vi "Teleop.vi"(10 "Match Info":T2={"Autonomous Elapsed Seconds"=0.0, "TeleOp Elapsed Seconds"=0.0, "Disabled Elapsed Seconds"=0.0, "Visited Autonomous"=FALSE, "Visited TeleOp"=FALSE, "Visited Disabled"=FALSE, "Autonomous Settings"={"Autonomous Style"=enum."Independent", "VI Refnum"=refnum}}, 11 "Call Context":T3) -> ()   [LabVIEW 2016]
doc: "This VI is called for each TeleOp packet received from the DS where the robot is not disabled. It is often used to read from the joysticks and update I/O or to update setpoints for timed control loops. It should complete and return within 20 milliseconds or it may miss DS packets."
uses:
  <vilib>/Rock Robotics/WPI/DriverStation/WPI_DriverStationDerivedRobotMode.ctl
  <vilib>/Rock Robotics/WPI/DriverStation/WPI_DriverStationMatch Info.ctl
  <vilib>/Rock Robotics/WPI/ThirdParty/CanMotor/TalonSRX/WPI_CANTalonSRX_BrakeOverride.ctl
  <vilib>/Rock Robotics/WPI/Utilities/WPI_GetSetVariantRefNum.vi
  <vilib>/Rock Robotics/Network Tables/NT Write Boolean Array.vi
  <vilib>/Rock Robotics/Network Tables/NT Write Numeric Array.vi
  <vilib>/Rock Robotics/Network Tables/NT Read Boolean.vi
  <vilib>/Rock Robotics/Network Tables/NT Read Number.vi
panel:
  in  "Output":dbl=0.5 format="%#_13g"
  in  "Reverse Soft Limit 2":dbl
  in  "Forward Soft Limit  2":dbl
  in  "Voltage Ramp Rate":dbl
  in  "Brake / Coast Mode":T1
  out "Brake Enabled":bool
  out "Reverse Soft Limit":bool
  out "Forward Soft Limit":bool
  out "Encoder V":dbl
  out "Battery Voltage":dbl
  out "Current":dbl
  out "Applied Throttle":dbl
  out "Sample Slider 0":dbl(slide) scale=0.0..5.0
  out "Sample Boolean 1":bool
  out "Sample Boolean 0":bool
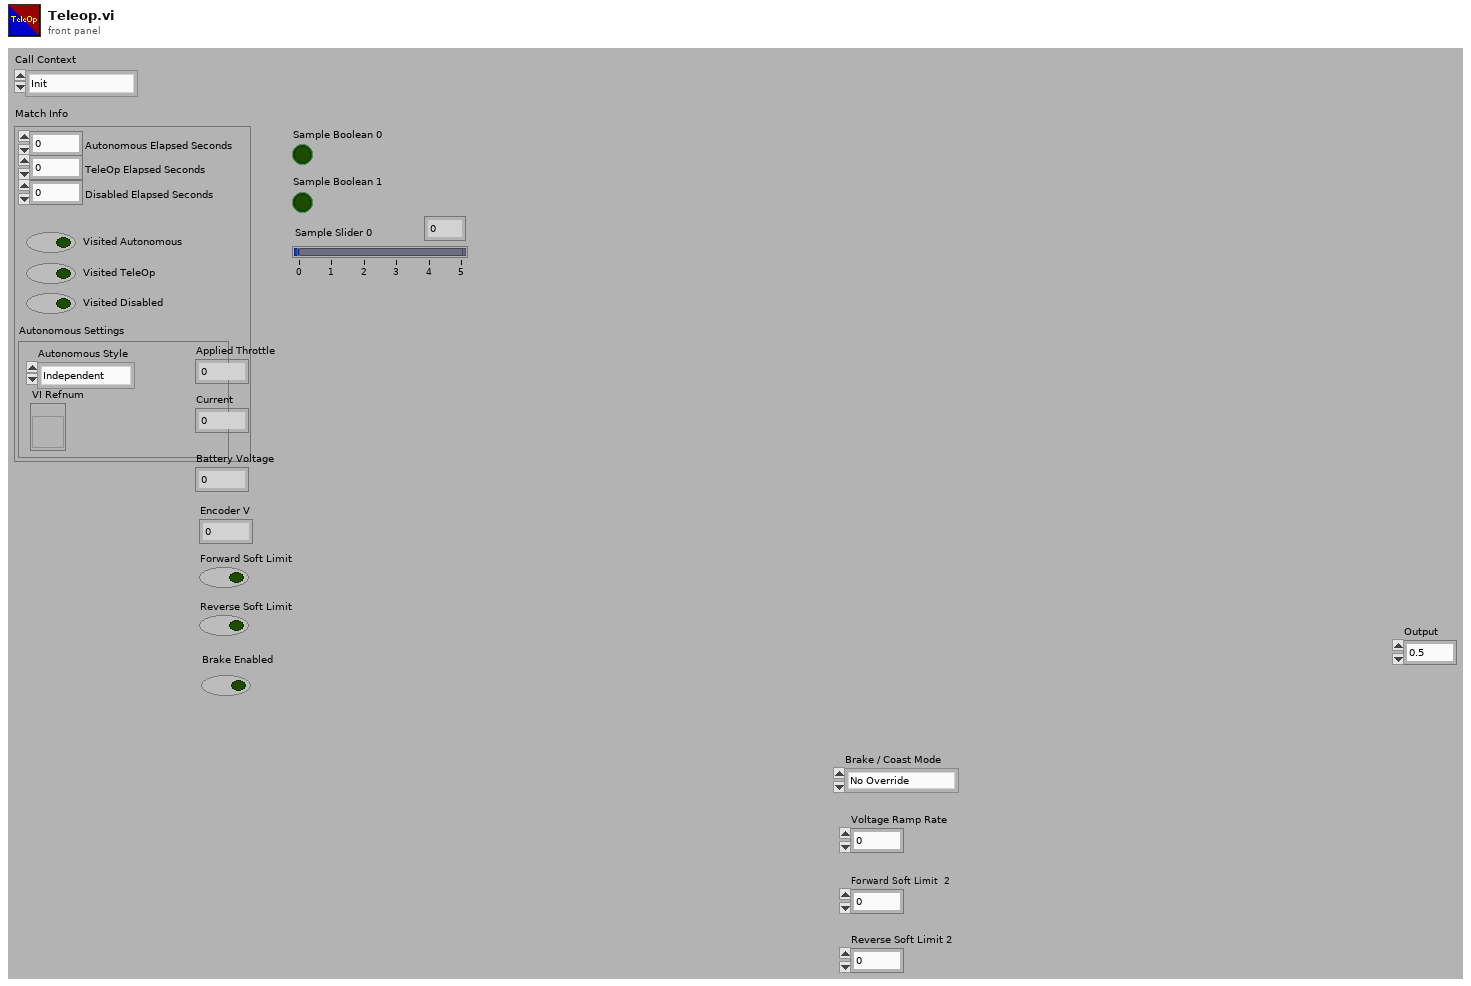
[diagram p1: front panel]
types:
  T1 = typedef "WPI_CANTalonSRX_BrakeOverride.ctl" = enum8{"No Override", "Override to Coast", "Override to Brake"}
  T2 = typedef "WPI_DriverStationMatch Info.ctl" = cluster{"Autonomous Elapsed Seconds":dbl, "TeleOp Elapsed Seconds":dbl, "Disabled Elapsed Seconds":dbl, "Visited Autonomous":bool, "Visited TeleOp":bool, "Visited Disabled":bool, "Autonomous Settings":cluster{"Autonomous Style":enum16{"Iterative", "Independent"}, "VI Refnum":refnum<vi>}}
  T3 = typedef "WPI_DriverStationDerivedRobotMode.ctl" = enum16{"Init", "Execute", "Stop"}
  T4 = typedef "WPI_RobotDriveDevRef.ctl" = cluster{"DevStatus":errorcluster, "Motors[]":T5[], "Square Inputs":bool, "Max Output":dbl}
  T5 = typedef "WPI_MotorControlDeviceRef.ctl" = cluster{"DeviceStatus":errorcluster, "Type":T6, "PWM":cluster{"PWM Channel":T7, "DeadBand":T8}, "CAN":cluster{"Device Number":u8, "SetOutput VI Ref":variant, "GetOutput VI Ref":variant, "Enable VI Ref":variant, "Disable VI Ref":variant, "Data":variant}, "Invert":bool}
  T6 = typedef "WPI_MotorControlType.ctl" = enum16{"PWM", "CAN"}
  T7 = typedef "FPGA_DIOPWMChannel.ctl" = enum8{"PWM 0", "PWM 1", "PWM 2", "PWM 3", "PWM 4", "PWM 5", "PWM 6", "PWM 7", "PWM 8", "PWM 9", "PWM MXP 0", "PWM MXP 1", "PWM MXP 2", "PWM MXP 3", "PWM MXP 4", "PWM MXP 5", "PWM MXP 6", "PWM MXP 7", "PWM MXP 8", "PWM MXP 9", "Invalid"}
  T8 = typedef "WPI_PWMDeadband.ctl" = cluster{"Name":string, "maxPositivePwm":i32, "minPositivePwm":i32, "centerPwm":i32, "maxNegativePwm":i32, "minNegativePwm":i32, "angularRange":u16}
  T9 = typedef "WPI_JoystickDevRef.ctl" = cluster{"Device":T10}
  T10 = typedef "WPI_JoystickDeviceEnum.ctl" = enum16{"USB 0", "USB 1", "USB 2", "USB 3", "USB 4", "USB 5"}
  T11 = typedef "WPI_CANTalonSRX_GlobalStatus.ctl" = cluster{"Applied Throttle":dbl, "Module Enabled":bool, "CAN Error":errorcluster, "Closed Loop Error":dbl, "Forward Limit Switch Closed":bool, "Reverse Limit Switch Closed":bool, "Sensor Position":dbl, "Sensor Velocity":dbl, "Current":dbl, "Sticky Fault - Over Temp":bool, "Sticky Fault - Under Voltage":bool, "Sticky Fault - Forward Limit":bool, "Sticky Fault - Reverse Limit":bool, "Sticky Fault - Forward Soft Limit":bool, "Sticky Fault - Reverse Soft Limit":bool, "Brake is Enabled":bool, "Encoder Position":dbl, "Encoder Velocity":dbl, "Encoder Index Count":dbl, "Encoder A Pin State":bool, "Encoder B Pin State":bool, "Encoder Index Pin State":bool, "Analog In":dbl, "Analog In Velocity":dbl, "Temperature (C)":dbl, "Battery Voltage":dbl, "Control 5 Is Supported":bool, "Current Profile Slot Select":dbl, "Pos Div 8":bool, "Vel Div 4":bool, "Pulse Width Position":i32, "Pulse Width Velocity":i32, "Pulse Width Rise To Rise (us)":i32, "Pulse Width Rise To Fall (us)":i32, "Mot Prof Active Is Under Run":bool, "Mot Prof Active Has Under Run":bool, "Mot Prof Active Is Last":bool, "Mot Prof Active Velocity Only":bool, "Mot Prof Active Is Valid":bool, "Mot Prof Buffer Is Full":bool, "Mot Prof Active Profile Slot Select":i32, "Mot Prof NextID":i32, "Mot Prof Count":i32, "Mot Prof Active Velocity":dbl, "Mot Prof Active Position":dbl, "Mot Prof Output Enable":i32}
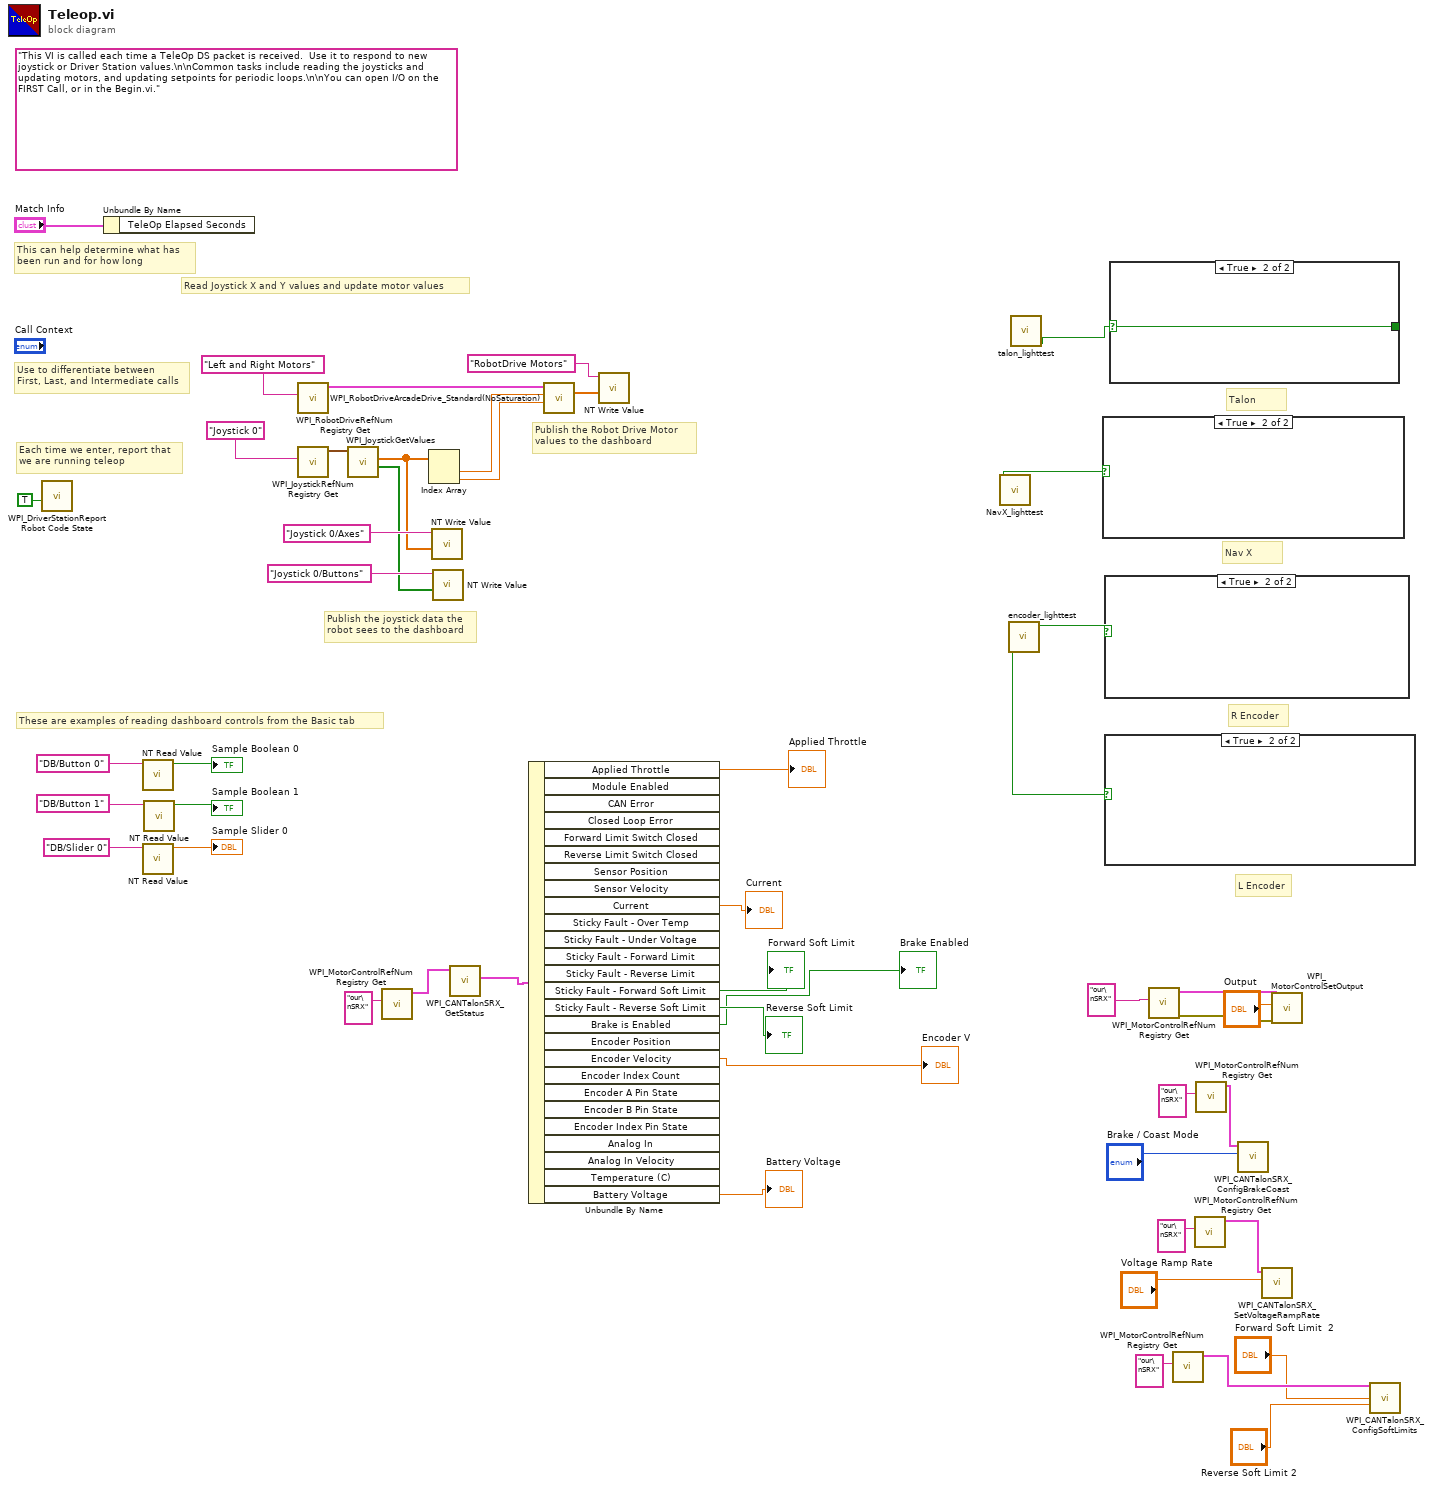
[diagram p0: block diagram]
diagram:
  (unwired) "This VI is called each time a TeleOp DS packet is received.  Use it to respond to new joystick or Driver Station values.\n\nCommon tasks include reading the joysticks and updating motors, and updating setpoints for periodic loops.\n\nYou can open I/O on the FIRST Call, or in the Begin.vi."
  # "Talon"
  # "Nav X"
  # "R Encoder"
  # "L Encoder"
  # "These are examples of reading dashboard controls from the Basic tab"
  # "Publish the Robot Drive Motor\nvalues to the dashboard"
  # "Publish the joystick data the\nrobot sees to the dashboard"
  # "Each time we enter, report that\nwe are running teleop"
  # "Use to differentiate between\nFirst, Last, and Intermediate calls"
  # "This can help determine what has\nbeen run and for how long"
  # "Read Joystick X and Y values and update motor values"
  n1 = call <vilib>:"WPI_DriverStationReport Robot Code State.vi"("TeleOp"=TRUE ("Autonomous")) -> ()  [unwired: 10 in, 1 out]
  n2 = Unbundle By Name("Match Info") -> ()  [unwired: 1 out]
  n3 = call-poly <vilib>:"NT Read Value.vi"("Name"="DB/Button 0" ("refnum name")) -> ("Boolean"=→"Sample Boolean 0":bool)  [unwired: 9 in, 1 out]
  n4 = call-poly <vilib>:"NT Read Value.vi"("Name"="DB/Slider 0" ("refnum name")) -> ("Numeric"=→"Sample Slider 0":dbl)  [unwired: 9 in, 1 out]
  n5 = call-poly <vilib>:"NT Read Value.vi"("Name"="DB/Button 1" ("refnum name")) -> ("Boolean"=→"Sample Boolean 1":bool)  [unwired: 9 in, 1 out]
  n6 = call <vilib>:"WPI_RobotDriveRefNum Registry Get.vi"("refnum name"="Left and Right Motors") -> ("RobotDriveDevRef"=w46:T4)  [unwired: 1 in, 9 out]
  n7 = call <vilib>:"WPI_JoystickRefNum Registry Get.vi"("refnum name"="Joystick 0") -> ("JoystickDevRef"=w43:T9)  [unwired: 1 in, 9 out]
  n8 = call <vilib>:"WPI_JoystickGetValues.vi"("JoystickDevRef"=w43) -> ("Buttons"=w37:bool[], "Axes"=w38:dbl[])  [unwired: 6 in, 3 out]
  n9 = call <vilib>:"WPI_MotorControlRefNum Registry Get.vi"("refnum name"="our\nSRX") -> ("MotorControlDevRef"=w18:T5)  [unwired: 9 in, 1 out]
  n10 = Index Array(array=w38) -> (element #1=w45:dbl, element #2=w41:dbl)  [unwired: 2 in]
  n11 = call-poly <vilib>:"NT Write Value.vi"("Numeric Array"=w38, "Name"="Joystick 0/Axes") -> ()  [unwired: 9 in, 1 out]
  n12 = call-poly <vilib>:"NT Write Value.vi"("Boolean Array"=w37, "Name"="Joystick 0/Buttons") -> ()  [unwired: 9 in, 1 out]
  n13 = call <vilib>:"WPI_CANTalonSRX_GetStatus.vi"("CAN Talon SRX Ref"=w18) -> ("Talon SRX Status"=w17:T11)  [unwired: 8 in, 2 out]
  n14 = Unbundle By Name(w17) -> ("Applied Throttle"=→"Applied Throttle":dbl, "Current"=→"Current":dbl, "Sticky Fault - Forward Soft Limit"=→"Forward Soft Limit":bool, "Sticky Fault - Reverse Soft Limit"=→"Reverse Soft Limit":bool, "Brake is Enabled"=→"Brake Enabled":bool, "Encoder Velocity"=→"Encoder V":dbl, "Battery Voltage"=→"Battery Voltage":dbl)  [unwired: 19 out]
  n15 = call <vilib>:"WPI_RobotDriveArcadeDrive_Standard(NoSaturation).vi"("Y axis value"=w41, "X axis value"=w45, "RobotDriveDevRef"=w46) -> ("Motor Values"=w30:dbl[])  [unwired: 1 in, 7 out]
  n16 = call-poly <vilib>:"NT Write Value.vi"("Numeric Array"=w30, "Name"="RobotDrive Motors") -> ()  [unwired: 9 in, 1 out]
  n17 = call "NavX_lighttest.vi"() -> ("NavX_test"=w27:bool)  [unwired: 11 in]
  n18 = call "encoder_lighttest.vi"() -> ("R Encoder"=w25:bool, "L Encoder"=w26:bool)  [unwired: 10 in]
  n19 = call "talon_lighttest.vi"() -> ("Boolean"=w28:bool)  [unwired: 11 in]
  n20 = case shown="True" w27 {
    frame False {
    }
    frame True {
    }
  }
  n21 = case shown="True" w25 {
    frame False {
    }
    frame True {
    }
  }
  n22 = case shown="True" w26 {
    frame False {
    }
    frame True {
    }
  }
  n23 = case shown="True" w28 {
    selector: w28 -> [w49 w50]
    tunnel: [w49 w50] -> _
    frame False {
    }
    frame True {
    }
  }
  n24 = call <vilib>:"WPI_MotorControlRefNum Registry Get.vi"("refnum name"="our\nSRX") -> ("error out"=w3:errorcluster, "MotorControlDevRef"=w2:T5)  [unwired: 9 in]
  n25 = call <vilib>:"WPI_MotorControlRefNum Registry Get.vi"("refnum name"="our\nSRX") -> ("MotorControlDevRef"=w7:T5)  [unwired: 9 in, 1 out]
  n26 = call <vilib>:"WPI_MotorControlRefNum Registry Get.vi"("refnum name"="our\nSRX") -> ("MotorControlDevRef"=w10:T5)  [unwired: 9 in, 1 out]
  n27 = call <vilib>:"WPI_MotorControlRefNum Registry Get.vi"("refnum name"="our\nSRX") -> ("MotorControlDevRef"=w13:T5)  [unwired: 9 in, 1 out]
  n28 = call <vilib>:"WPI_CANTalonSRX_ConfigBrakeCoast.vi"("Brake / Coast Mode"="Brake / Coast Mode", "CAN Talon SRX Ref"=w13) -> ()  [unwired: 8 in, 2 out]
  n29 = call <vilib>:"WPI_CANTalonSRX_SetVoltageRampRate.vi"("Throttle Ramp Rate (percent/s)"="Voltage Ramp Rate", "CAN Talon SRX Ref"=w10) -> ()  [unwired: 8 in, 2 out]
  n30 = call <vilib>:"WPI_MotorControlSetOutput.vi"("error in (no error)"=w3, "Output"="Output", "MotorControlDevRef"=w2) -> ()  [unwired: 6 in, 3 out]
  n31 = call <vilib>:"WPI_CANTalonSRX_ConfigSoftLimits.vi"("CAN Talon SRX Ref"=w7, "Forward Limit Position"="Forward Soft Limit  2", "Reverse Limit Position"="Reverse Soft Limit 2") -> ()  [unwired: 11 in, 2 out]
